vi "Launch Root Panel Window.vi"(5 "Window Position (Maximize First Call)":refnum<class "Window Position.lvclass">, 6 "timeout in ms (-1)":i32=-1, 7 "Autoshow? (T)":bool=TRUE, 8 "Error In":errorcluster, 10 "Title":string, 11 "Panel Actor in":refnum<class "Panel Actor.lvclass">) -> (0 "Error Out":errorcluster, 2 "Actor's Enqueuer":refnum<class "Message Enqueuer.lvclass">)   [LabVIEW 2019, in "Panel Actor.lvlib" / "Panel Actor.lvclass"]
doc: "Launches a Root Panel using the window Panel type.\n\n<B>Panel Actor In:</B> Panel Actor object to launch\n<B>Title:</B> Sets the default title for the window.\n<B>Autoshow?</B> If Autoshow? is TRUE, then the Window will be displayed on initialization. If it is FALSE, then the Show method must be called manually.\n<B>Window Position:</B> Window Position object to control window position behavior.\n<B>timeout in ms</B> Time to wait for the panel to initialize\n<B>Error In:</B> Describes error conditions that occur before this node runs.\n\n<B>Actor's Enqueuer:</B> Enqueuer for newly spawned actor\n<B>Error Out:</B> Contains error information.\n----\nPlease see the following web address for additional documentation and tutorial information:\nhttp://www.mooregoodideas.com/mgi-panel-manager/\n\nAuthor: Derek Trepanier\n\nCopyright (c) 2018, Moore Good Ideas, Inc.\n\nAll rights reserved.\n\nRedistribution and use in source and binary forms, with or without modification, are permitted provided that the following conditions are met:\n\n * Redistributions of source code must retain the above copyright notice, this list of conditions and the following disclaimer.\n * Redistributions in binary form must reproduce the above copyright notice, this list of conditions and the following disclaimer in the documentation and/or other materials provided with the distribution.\n * Neither the name of Moore Good Ideas, Inc. nor the names of its contributors may be used to endorse or promote products derived from this software without specific prior written permission.\n\nTHIS SOFTWARE IS PROVIDED BY THE COPYRIGHT HOLDERS AND CONTRIBUTORS \"AS IS\" AND ANY EXPRESS OR IMPLIED WARRANTIES, INCLUDING, BUT NOT LIMITED TO, THE IMPLIED WARRANTIES OF MERCHANTABILITY AND FITNESS FOR A PARTICULAR PURPOSE ARE DISCLAIMED. IN NO EVENT SHALL THE COPYRIGHT OWNER OR CONTRIBUTORS BE LIABLE FOR ANY DIRECT, INDIRECT, INCIDENTAL, SPECIAL, EXEMPLARY, OR CONSEQUENTIAL DAMAGES (INCLUDING, BUT NOT LIMITED TO, PROCUREMENT OF SUBSTITUTE GOODS OR SERVICES; LOSS OF USE, DATA, OR PROFITS; OR BUSINESS INTERRUPTION) HOWEVER CAUSED AND ON ANY THEORY OF LIABILITY, WHETHER IN CONTRACT, STRICT LIABILITY, OR TORT (INCLUDING NEGLIGENCE OR OTHERWISE) ARISING IN ANY WAY OUT OF THE USE OF THIS SOFTWARE, EVEN IF ADVISED OF THE POSSIBILITY OF SUCH DAMAGE."
uses:
  Panel Actor.lvclass
  builds/Engine/Panel.lvlibp
  builds/Engine/Panel.lvlibp/Panel/Window/Window.vi
  builds/Engine/Panel.lvlibp/Panel/Window/Window.lvclass
  builds/Engine/Panel.lvlibp/Window Position/Maximize/Maximize.lvclass
  builds/Engine/Panel.lvlibp/Window Position/Window Position.lvclass
  C:/Users/public/Documents/Development/builds/Engine/Panel.lvlibp/Window Position/Window Position.lvclass
  C:/Users/public/Documents/Development/builds/Engine/Panel.lvlibp/Panel/Panel.lvclass
  builds/Engine/Actor Framework.lvlibp/1abvi3w/vi.lib/ActorFramework/Message Enqueuer/Message Enqueuer.lvclass
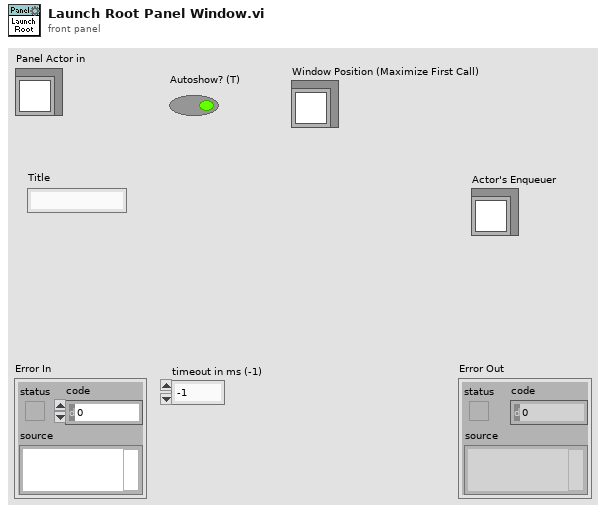
[diagram p1: front panel]
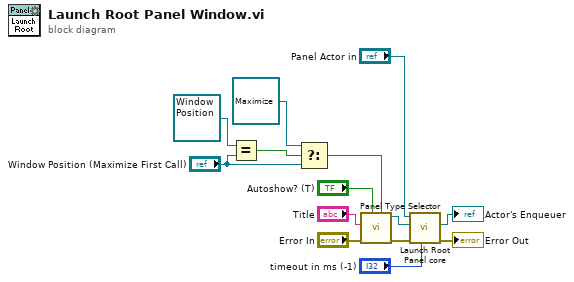
[diagram p0: block diagram]
diagram:
  n1 = Equal?(x=refnum<class "Window Position.lvclass"> refnum ("y"), y="Window Position (Maximize First Call)") -> (x = y?=w2:bool)
  n2 = Select(t=refnum<class "Maximize.lvclass"> refnum ("Panel.lvlibp:Maximize.lvclass"), s=w2, f="Window Position (Maximize First Call)") -> (s? t:f=w4:refnum<class "Window Position.lvclass">)
  n3 = call-poly "Panel Type Selector.vi"("Window Position"=w4, "Autoshow? (T)"="Autoshow? (T)", "error in (no error)"="Error In", "Default Title"="Title") -> ("error out"=w7:errorcluster, "Window out"=w8:refnum<class "Window.lvclass">)  [unwired: 6 in]
  n4 = call "Launch Root Panel core.vi"("timeout in ms (-1)"="timeout in ms (-1)", "Error In"=w7, "Panel"=w8, "Panel Actor in"="Panel Actor in") -> ("Error Out"=→"Error Out":errorcluster, "Actor's Enqueuer"=→"Actor's Enqueuer":refnum<class "Message Enqueuer.lvclass">)  [unwired: 6 in]
